vi "getMultiChannelsVoltage.vi"(6 "测试时断开电源？":bool=TRUE, 8 "调试？T/F":bool=TRUE, 9 "传感器数目":i32=1, 10 "控制板":refnum<visa-resource-name>, 11 "电压表":refnum<visa-resource-name>) -> (3 "获取结果":string[](array[string]))   [LabVIEW 2017]
uses:
  <vilib>/Instr/_visa.llb/VISA Configure Serial Port (Instr).vi
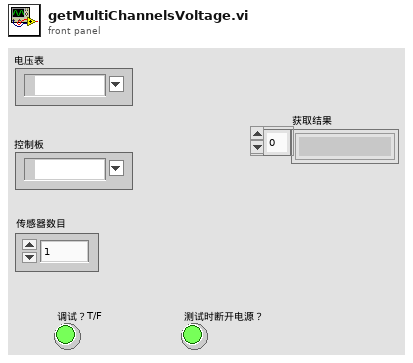
[diagram p1: front panel]
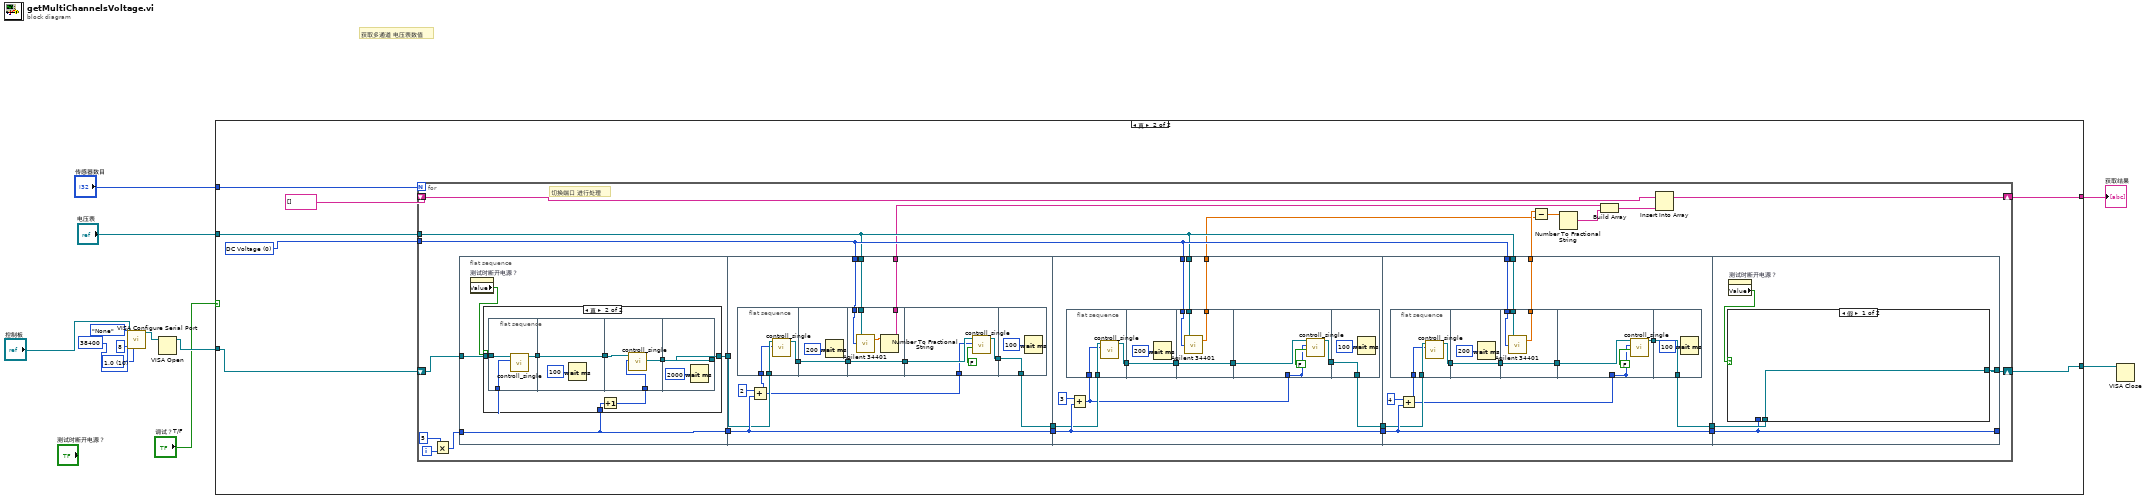
[diagram p0: block diagram]
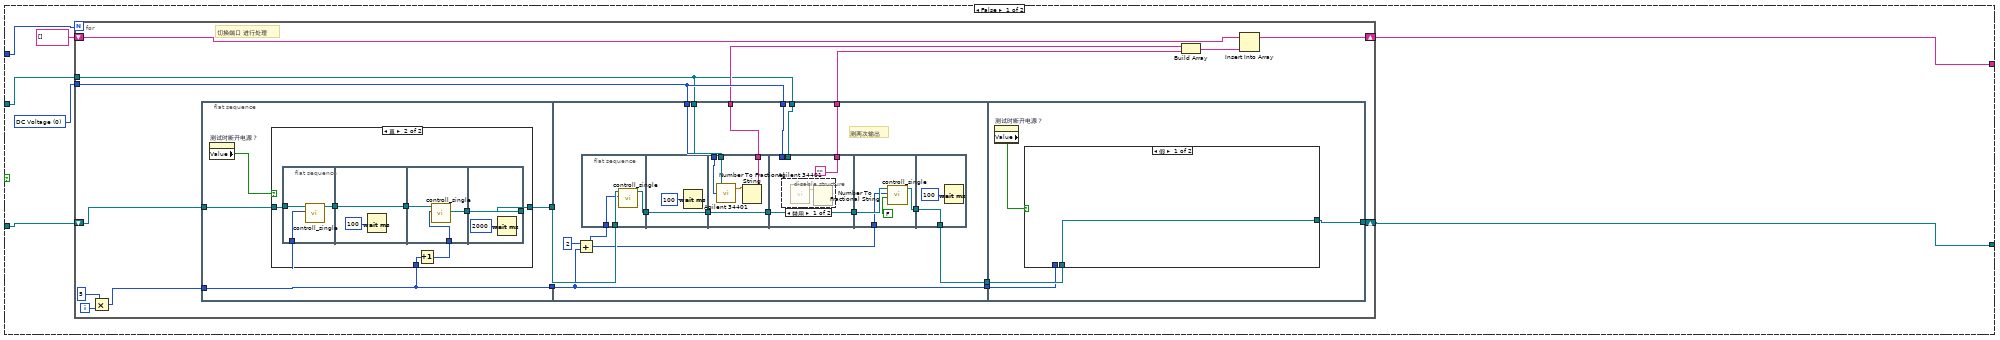
[diagram p2: hidden frame]
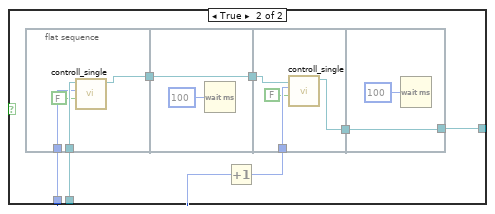
[diagram p5: hidden frame]
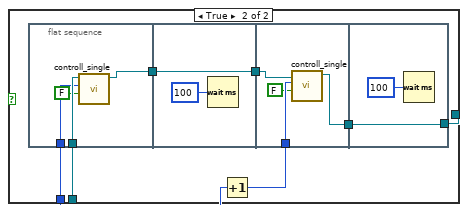
[diagram p7: hidden frame]
diagram:
  w3 = u16 10 items=["1.0"=10, "1.5"=15, "2.0"=20] ("stop bits (10: 1 bit)")
  # "获取多通道 电压表数值"
  n1 = call-poly "VISA Configure Serial Port"("VISA resource name"="控制板", "baud rate (9600)"=u32 38400, "data bits (8)"=u16 8, "parity (0:none)"=enum16{"None", "Odd", "Even", "Mark", "Space"}."None", "stop bits (10: 1 bit)"=w3) -> ("VISA resource name out"=w7:refnum<visa-resource-name>)  [unwired: 9 in, 1 out]
  n2 = VISA Open(VISA resource name=w7) -> (VISA resource name=w2:refnum<visa-resource-name>)  [unwired: 4 in, 1 out]
  n3 = case shown="真" "调试？T/F" {
    tunnel: "电压表" -> [w18 w122]
    tunnel: "传感器数目" -> [w17 w121]
    tunnel: [w13 w119] -> w10
    tunnel: [w14 w118] -> w9
    tunnel: w2 -> [w16 w117]
    frame False {
      w15 = u16 0 items=["DC Voltage", "AC Voltage", "2 - Wire Resistance", "4 - Wire Resistance", "DC Current", "AC Current", "Frequency", "Period", "Continuity", "Diode Checking", "VDC:VDC Ratio", "Temperature", "Capacitance"] ("Function (0: DC Voltage)")
      n4 = for {
        N: w17 -> [_]
        tunnel: w18 -> [w21]
        tunnel: w15 -> [w29]
        shift-right: [w27] -> w14
        shift-left: w16 -> [w26]
        shift-right: [w24] -> w13
        shift-left: string[] [] -> [w23]
        i -> [w35]
        # "切换端口 进行处理"
        n5 = Multiply(x=5, y=w35) -> (x*y=w33:i32)
        n6 = flat-sequence {
          tunnel: [w39] -> w32
          tunnel: [w37] -> w31
          tunnel: w26 -> [w38]
          tunnel: w33 -> [w39]
          tunnel: [w63] -> w30
          tunnel: w29 -> [w59]
          tunnel: [w65] -> w28
          tunnel: w29 -> [w68]
          tunnel: w21 -> [w69]
          tunnel: w31 -> [w70]
          tunnel: w32 -> [w64]
          tunnel: [w64] -> w22
          tunnel: w21 -> [w60]
          tunnel: [w58] -> w20
          tunnel: w30 -> [w96]
          tunnel: [w94] -> w27
          tunnel: w22 -> [w95]
          frame #0 {
            n7 = property on="测试时断开电源？" class="Bool (严格)"() -> ("Value"=w36:bool)  [unwired: 2 in, 2 out]
            n8 = case shown="真" w36 {
              tunnel: w39 -> [_ w44]
              tunnel: w38 -> [w40 w43]
              tunnel: [w40 w42] -> w37
              frame False {
              }
              frame True {
                n9 = flat-sequence {
                  tunnel: w44 -> [w50]
                  tunnel: w43 -> [w48]
                  tunnel: [w49] -> w47
                  tunnel: w47 -> [w52]
                  tunnel: [w52] -> w46
                  tunnel: w46 -> [w55]
                  tunnel: w41 -> [w53]
                  tunnel: [w54] -> w45
                  tunnel: [w57] -> w42
                  tunnel: w45 -> [w57]
                  frame #0 {
                    n10 = call "controll_single.vi"("控制编号"=w50, "VISA资源名称"=w48) -> ("VISA资源名称输出"=w49:refnum<visa-resource-name>)  [unwired: 9 in]
                  }
                  frame #1 {
                    n11 = Wait (ms)(milliseconds to wait=u32 100 ("等待时间（毫秒）")) -> ()  [unwired: 1 out]
                  }
                  frame #2 {
                    n12 = call "controll_single.vi"("控制编号"=w53, "VISA资源名称"=w55) -> ("VISA资源名称输出"=w54:refnum<visa-resource-name>)  [unwired: 9 in]
                  }
                  frame #3 {
                    n13 = Wait (ms)(milliseconds to wait=u32 2000 ("等待时间（毫秒）")) -> ()  [unwired: 1 out]
                  }
                }
                n14 = Increment(x=w44) -> (x+1=w41:i32)
              }
            }
          }
          frame #1 {
            # "测两次输出"
            n15 = Add(x=2, y=w64) -> (x+y=w66:i32)
            n16 = flat-sequence {
              tunnel: w70 -> [w76]
              tunnel: w66 -> [w75]
              tunnel: [w74] -> w73
              tunnel: [w77] -> w72
              tunnel: w73 -> [w77]
              tunnel: w69 -> [w82]
              tunnel: w68 -> [w81]
              tunnel: [w80] -> w62
              tunnel: w72 -> [w80]
              tunnel: [w79] -> w65
              tunnel: w62 -> [w85]
              tunnel: [w85] -> w61
              tunnel: w60 -> [_]
              tunnel: w59 -> [_]
              tunnel: [""] -> w58
              tunnel: w66 -> [w89]
              tunnel: w61 -> [w90]
              tunnel: [w87] -> w71
              tunnel: w71 -> [w91]
              tunnel: [w91] -> w63
              frame #0 {
                n17 = call "controll_single.vi"("控制编号"=w75, "VISA资源名称"=w76) -> ("VISA资源名称输出"=w74:refnum<visa-resource-name>)  [unwired: 9 in]
              }
              frame #1 {
                n18 = Wait (ms)(milliseconds to wait=u32 100 ("等待时间（毫秒）")) -> ()  [unwired: 1 out]
              }
              frame #2 {
                n19 = call "Agilent 34401.vi"("Function (0: DC Voltage)"=w81, "VISA resource name"=w82) -> ("Measurement"=w83:dbl)  [unwired: 1 in, 1 out]
                n20 = Number To Fractional String(number=w83) -> (F-format string=w79:string)  [unwired: 3 in]
              }
              frame #3 {
                n21 = disable-structure shown="禁用" {
                  frame Disabled {
                    n22 = call "Agilent 34401.vi"() -> ("Measurement"=w86:dbl)  [unwired: 3 in, 1 out]
                    n23 = Number To Fractional String(number=w86) -> ()  [unwired: 3 in, 1 out]
                  }
                  frame Enabled {
                  }
                }
              }
              frame #4 {
                n24 = call "controll_single.vi"("开关"=FALSE, "控制编号"=w89, "VISA资源名称"=w90) -> ("VISA资源名称输出"=w87:refnum<visa-resource-name>)  [unwired: 8 in]
              }
              frame #5 {
                n25 = Wait (ms)(milliseconds to wait=u32 100 ("等待时间（毫秒）")) -> ()  [unwired: 1 out]
              }
            }
          }
          frame #2 {
            n26 = property on="测试时断开电源？" class="Bool (严格)"() -> ("Value"=w93:bool)  [unwired: 2 in, 2 out]
            n27 = case shown="假" w93 {
              tunnel: w96 -> [w97 w101]
              tunnel: w95 -> [_ w100]
              tunnel: [w97 w98] -> w94
              frame False {
              }
              frame True {
                n28 = flat-sequence {
                  tunnel: w101 -> [w108]
                  tunnel: w100 -> [w107]
                  tunnel: [w105] -> w104
                  tunnel: [w109] -> w103
                  tunnel: w104 -> [w109]
                  tunnel: w103 -> [w114]
                  tunnel: w99 -> [w113]
                  tunnel: [w111] -> w102
                  tunnel: w102 -> [w115]
                  tunnel: [w115] -> w98
                  frame #0 {
                    n29 = call "controll_single.vi"("开关"=FALSE, "控制编号"=w107, "VISA资源名称"=w108) -> ("VISA资源名称输出"=w105:refnum<visa-resource-name>)  [unwired: 8 in]
                  }
                  frame #1 {
                    n30 = Wait (ms)(milliseconds to wait=u32 100 ("等待时间（毫秒）")) -> ()  [unwired: 1 out]
                  }
                  frame #2 {
                    n31 = call "controll_single.vi"("开关"=FALSE, "控制编号"=w113, "VISA资源名称"=w114) -> ("VISA资源名称输出"=w111:refnum<visa-resource-name>)  [unwired: 8 in]
                  }
                  frame #3 {
                    n32 = Wait (ms)(milliseconds to wait=u32 100 ("等待时间（毫秒）")) -> ()  [unwired: 1 out]
                  }
                }
                n33 = Increment(x=w100) -> (x+1=w99:i32)
              }
            }
          }
        }
        n34 = Build Array(w28, w20) -> (w25:string[])
        n35 = Insert Into Array(array=w23, new element=w25) -> (w24:string[])  [unwired: 1 in]
      }
    }
    frame True {
      w123 = u16 0 items=["DC Voltage", "AC Voltage", "2 - Wire Resistance", "4 - Wire Resistance", "DC Current", "AC Current", "Frequency", "Period", "Continuity", "Diode Checking", "VDC:VDC Ratio", "Temperature", "Capacitance"] ("Function (0: DC Voltage)")
      n36 = for {
        N: w121 -> [_]
        tunnel: w122 -> [w134]
        tunnel: w123 -> [w135]
        shift-right: [w128] -> w118
        shift-left: w117 -> [w127]
        shift-right: [w125] -> w119
        shift-left: string[] [] -> [w124]
        i -> [w146]
        # "切换端口 进行处理"
        n37 = Multiply(x=5, y=w146) -> (x*y=w144:i32)
        n38 = flat-sequence {
          tunnel: [w150] -> w143
          tunnel: [w148] -> w142
          tunnel: w127 -> [w149]
          tunnel: w144 -> [w150]
          tunnel: w143 -> [w180]
          tunnel: w142 -> [w179]
          tunnel: [w180] -> w141
          tunnel: [w170] -> w140
          tunnel: w134 -> [w178]
          tunnel: w135 -> [w177]
          tunnel: [w169] -> w130
          tunnel: w141 -> [w202]
          tunnel: w140 -> [w201]
          tunnel: w134 -> [w204]
          tunnel: w135 -> [w203]
          tunnel: [w202] -> w139
          tunnel: [w198] -> w138
          tunnel: [w197] -> w132
          tunnel: w139 -> [w231]
          tunnel: w138 -> [w230]
          tunnel: [w231] -> w137
          tunnel: [w225] -> w136
          tunnel: w135 -> [w229]
          tunnel: w134 -> [w228]
          tunnel: [w224] -> w133
          tunnel: [w253] -> _
          tunnel: w137 -> [w253]
          tunnel: w136 -> [w254]
          tunnel: [w252] -> w128
          frame #0 {
            n39 = property on="测试时断开电源？" class="Bool (严格)"() -> ("Value"=w147:bool)  [unwired: 2 in, 2 out]
            n40 = case shown="真" w147 {
              tunnel: w150 -> [_ w155]
              tunnel: w149 -> [w151 w154]
              tunnel: [w151 w153] -> w148
              frame False {
              }
              frame True {
                n41 = flat-sequence {
                  tunnel: w155 -> [w161]
                  tunnel: w154 -> [w159]
                  tunnel: [w160] -> w158
                  tunnel: w158 -> [w163]
                  tunnel: [w163] -> w157
                  tunnel: w157 -> [w166]
                  tunnel: w152 -> [w164]
                  tunnel: [w165] -> w156
                  tunnel: [w168] -> w153
                  tunnel: w156 -> [w168]
                  frame #0 {
                    n42 = call "controll_single.vi"("控制编号"=w161, "VISA资源名称"=w159) -> ("VISA资源名称输出"=w160:refnum<visa-resource-name>)  [unwired: 9 in]
                  }
                  frame #1 {
                    n43 = Wait (ms)(milliseconds to wait=u32 100 ("等待时间（毫秒）")) -> ()  [unwired: 1 out]
                  }
                  frame #2 {
                    n44 = call "controll_single.vi"("控制编号"=w164, "VISA资源名称"=w166) -> ("VISA资源名称输出"=w165:refnum<visa-resource-name>)  [unwired: 9 in]
                  }
                  frame #3 {
                    n45 = Wait (ms)(milliseconds to wait=u32 2000 ("等待时间（毫秒）")) -> ()  [unwired: 1 out]
                  }
                }
                n46 = Increment(x=w155) -> (x+1=w152:i32)
              }
            }
          }
          frame #1 {
            n47 = flat-sequence {
              tunnel: w179 -> [w183]
              tunnel: w172 -> [w182]
              tunnel: [w181] -> w173
              tunnel: [w184] -> w174
              tunnel: w173 -> [w184]
              tunnel: w178 -> [w189]
              tunnel: w177 -> [w188]
              tunnel: [w187] -> w175
              tunnel: w174 -> [w187]
              tunnel: [w186] -> w169
              tunnel: w172 -> [w193]
              tunnel: w175 -> [w194]
              tunnel: [w191] -> w171
              tunnel: w171 -> [w195]
              tunnel: [w195] -> w170
              frame #0 {
                n48 = call "controll_single.vi"("控制编号"=w182, "VISA资源名称"=w183) -> ("VISA资源名称输出"=w181:refnum<visa-resource-name>)  [unwired: 9 in]
              }
              frame #1 {
                n49 = Wait (ms)(milliseconds to wait=u32 200 ("等待时间（毫秒）")) -> ()  [unwired: 1 out]
              }
              frame #2 {
                n50 = call "Agilent 34401.vi"("Function (0: DC Voltage)"=w188, "VISA resource name"=w189) -> ("Measurement"=w190:dbl)  [unwired: 1 in, 1 out]
                n51 = Number To Fractional String(number=w190) -> (F-format string=w186:string)  [unwired: 3 in]
              }
              frame #3 {
                n52 = call "controll_single.vi"("开关"=FALSE, "控制编号"=w193, "VISA资源名称"=w194) -> ("VISA资源名称输出"=w191:refnum<visa-resource-name>)  [unwired: 8 in]
              }
              frame #4 {
                n53 = Wait (ms)(milliseconds to wait=u32 100 ("等待时间（毫秒）")) -> ()  [unwired: 1 out]
              }
            }
            n54 = Add(x=2, y=w180) -> (x+y=w172:i32)
          }
          frame #2 {
            n55 = flat-sequence {
              tunnel: w201 -> [w211]
              tunnel: w200 -> [w210]
              tunnel: [w209] -> w208
              tunnel: [w212] -> w207
              tunnel: w208 -> [w212]
              tunnel: w204 -> [w217]
              tunnel: w203 -> [w216]
              tunnel: [w215] -> w206
              tunnel: w207 -> [w215]
              tunnel: [w214] -> w197
              tunnel: [w219] -> _
              tunnel: w206 -> [w221]
              tunnel: w200 -> [w219]
              tunnel: [w218] -> w199
              tunnel: w199 -> [w222]
              tunnel: [w222] -> w198
              frame #0 {
                n56 = call "controll_single.vi"("控制编号"=w210, "VISA资源名称"=w211) -> ("VISA资源名称输出"=w209:refnum<visa-resource-name>)  [unwired: 9 in]
              }
              frame #1 {
                n57 = Wait (ms)(milliseconds to wait=u32 200 ("等待时间（毫秒）")) -> ()  [unwired: 1 out]
              }
              frame #2 {
                n58 = call "Agilent 34401.vi"("Function (0: DC Voltage)"=w216, "VISA resource name"=w217) -> ("Measurement"=w214:dbl)  [unwired: 1 in, 1 out]
              }
              frame #3 {
                n59 = call "controll_single.vi"("开关"=FALSE, "控制编号"=w219, "VISA资源名称"=w221) -> ("VISA资源名称输出"=w218:refnum<visa-resource-name>)  [unwired: 8 in]
              }
              frame #4 {
                n60 = Wait (ms)(milliseconds to wait=u32 100 ("等待时间（毫秒）")) -> ()  [unwired: 1 out]
              }
            }
            n61 = Add(x=3, y=w202) -> (x+y=w200:i32)
          }
          frame #3 {
            n62 = flat-sequence {
              tunnel: w230 -> [w238]
              tunnel: w227 -> [w237]
              tunnel: [w236] -> w235
              tunnel: [w239] -> w234
              tunnel: w235 -> [w239]
              tunnel: w228 -> [w244]
              tunnel: w229 -> [w243]
              tunnel: [w242] -> w233
              tunnel: w234 -> [w242]
              tunnel: [w241] -> w224
              tunnel: w227 -> [w246]
              tunnel: w233 -> [w248]
              tunnel: [w246] -> _
              tunnel: [w245] -> w226
              tunnel: w226 -> [w249]
              tunnel: [w249] -> w225
              frame #0 {
                n63 = call "controll_single.vi"("控制编号"=w237, "VISA资源名称"=w238) -> ("VISA资源名称输出"=w236:refnum<visa-resource-name>)  [unwired: 9 in]
              }
              frame #1 {
                n64 = Wait (ms)(milliseconds to wait=u32 200 ("等待时间（毫秒）")) -> ()  [unwired: 1 out]
              }
              frame #2 {
                n65 = call "Agilent 34401.vi"("Function (0: DC Voltage)"=w243, "VISA resource name"=w244) -> ("Measurement"=w241:dbl)  [unwired: 1 in, 1 out]
              }
              frame #3 {
                n66 = call "controll_single.vi"("开关"=FALSE, "控制编号"=w246, "VISA资源名称"=w248) -> ("VISA资源名称输出"=w245:refnum<visa-resource-name>)  [unwired: 8 in]
              }
              frame #4 {
                n67 = Wait (ms)(milliseconds to wait=u32 100 ("等待时间（毫秒）")) -> ()  [unwired: 1 out]
              }
            }
            n68 = Add(x=4, y=w231) -> (x+y=w227:i32)
          }
          frame #4 {
            n69 = property on="测试时断开电源？" class="Bool (严格)"() -> ("Value"=w251:bool)  [unwired: 2 in, 2 out]
            n70 = case shown="假" w251 {
              tunnel: w254 -> [w255 w259]
              tunnel: w253 -> [_ w258]
              tunnel: [w255 w256] -> w252
              frame False {
              }
              frame True {
                n71 = flat-sequence {
                  tunnel: w259 -> [w266]
                  tunnel: w258 -> [w265]
                  tunnel: [w263] -> w262
                  tunnel: [w267] -> w261
                  tunnel: w262 -> [w267]
                  tunnel: w261 -> [w272]
                  tunnel: w257 -> [w271]
                  tunnel: [w269] -> w260
                  tunnel: w260 -> [w273]
                  tunnel: [w273] -> w256
                  frame #0 {
                    n72 = call "controll_single.vi"("开关"=FALSE, "控制编号"=w265, "VISA资源名称"=w266) -> ("VISA资源名称输出"=w263:refnum<visa-resource-name>)  [unwired: 8 in]
                  }
                  frame #1 {
                    n73 = Wait (ms)(milliseconds to wait=u32 100 ("等待时间（毫秒）")) -> ()  [unwired: 1 out]
                  }
                  frame #2 {
                    n74 = call "controll_single.vi"("开关"=FALSE, "控制编号"=w271, "VISA资源名称"=w272) -> ("VISA资源名称输出"=w269:refnum<visa-resource-name>)  [unwired: 8 in]
                  }
                  frame #3 {
                    n75 = Wait (ms)(milliseconds to wait=u32 100 ("等待时间（毫秒）")) -> ()  [unwired: 1 out]
                  }
                }
                n76 = Increment(x=w258) -> (x+1=w257:i32)
              }
            }
          }
        }
        n77 = Subtract(x=w133, y=w132) -> (x-y=w131:dbl)
        n78 = Number To Fractional String(number=w131) -> (F-format string=w129:string)  [unwired: 3 in]
        n79 = Build Array(w130, w129) -> (w126:string[])
        n80 = Insert Into Array(array=w124, new element=w126) -> (w125:string[])  [unwired: 1 in]
      }
    }
  }
  "获取结果" <- w10
  n81 = VISA Close(VISA resource name=w9) -> ()  [unwired: 1 in, 1 out]
